vi "Recall aNETka (single).vi"() -> ()   [LabVIEW 2010]
uses:
  <vilib>/Utility/file.llb/Read From Spreadsheet File (DBL).vi
panel:
  in  "Case Constant\n(See Context Help)":bool
  out "aNETka outputs":dbl[](array[numeric])=[10.998674392700195] format="%.4f"
  out "1D config":i32[](array[numeric])=[2, 5, 1]
  out "Function":enum16{"Linear", "Sigmoid", "Tangent hyp."}(ring)=enum."Sigmoid"
  out "aNETka config":i32[](array[numeric])=[2, 5, 1] min=0 max=100 step=1
  out "aNETka configuration":cluster{dbl[], dbl[]}[](graph)=[{[2.0, 3.0], [5.5, 3.5]}, {[2.0, 3.0], [4.5, 3.5]}, {[2.0, 3.0], [3.5, 3.5]}, {[2.0, 3.0], [2.5, 3.5]}, {[2.0, 3.0], [1.5, 3.5]}, {[1.0, 2.0], [4.0, 1.5]}, {[1.0, 2.0], [4.0, 2.5]}, {[1.0, 2.0], [4.0, 3.5]}, {[1.0, 2.0], [4.0, 4.5]}, {[1.0, 2.0], [4.0, 5.5]}, {[1.0, 2.0], [3.0, 1.5]}, {[1.0, 2.0], [3.0, 2.5]}, {[1.0, 2.0], [3.0, 3.5]}, {[1.0, 2.0], [3.0, 4.5]}, {[1.0, 2.0], [3.0, 5.5]}]
  # "Inputs"
  # "Outputs"
  # "(Hidden layers)"
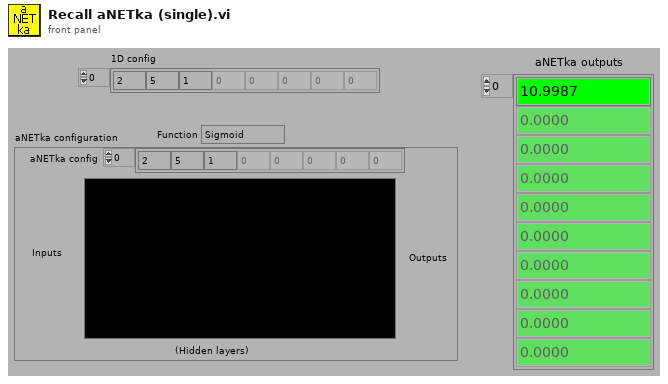
[diagram p1: front panel]
types:
  T1 = enum32{"existing file", "new file", "new or existing file", "existing dir", "new dir", "new or existing dir", "existing file (use LLBs)", "new file (use LLBs)", "new or existing file (use LLBs)", "new or existing file or directory (use LLBs)"}
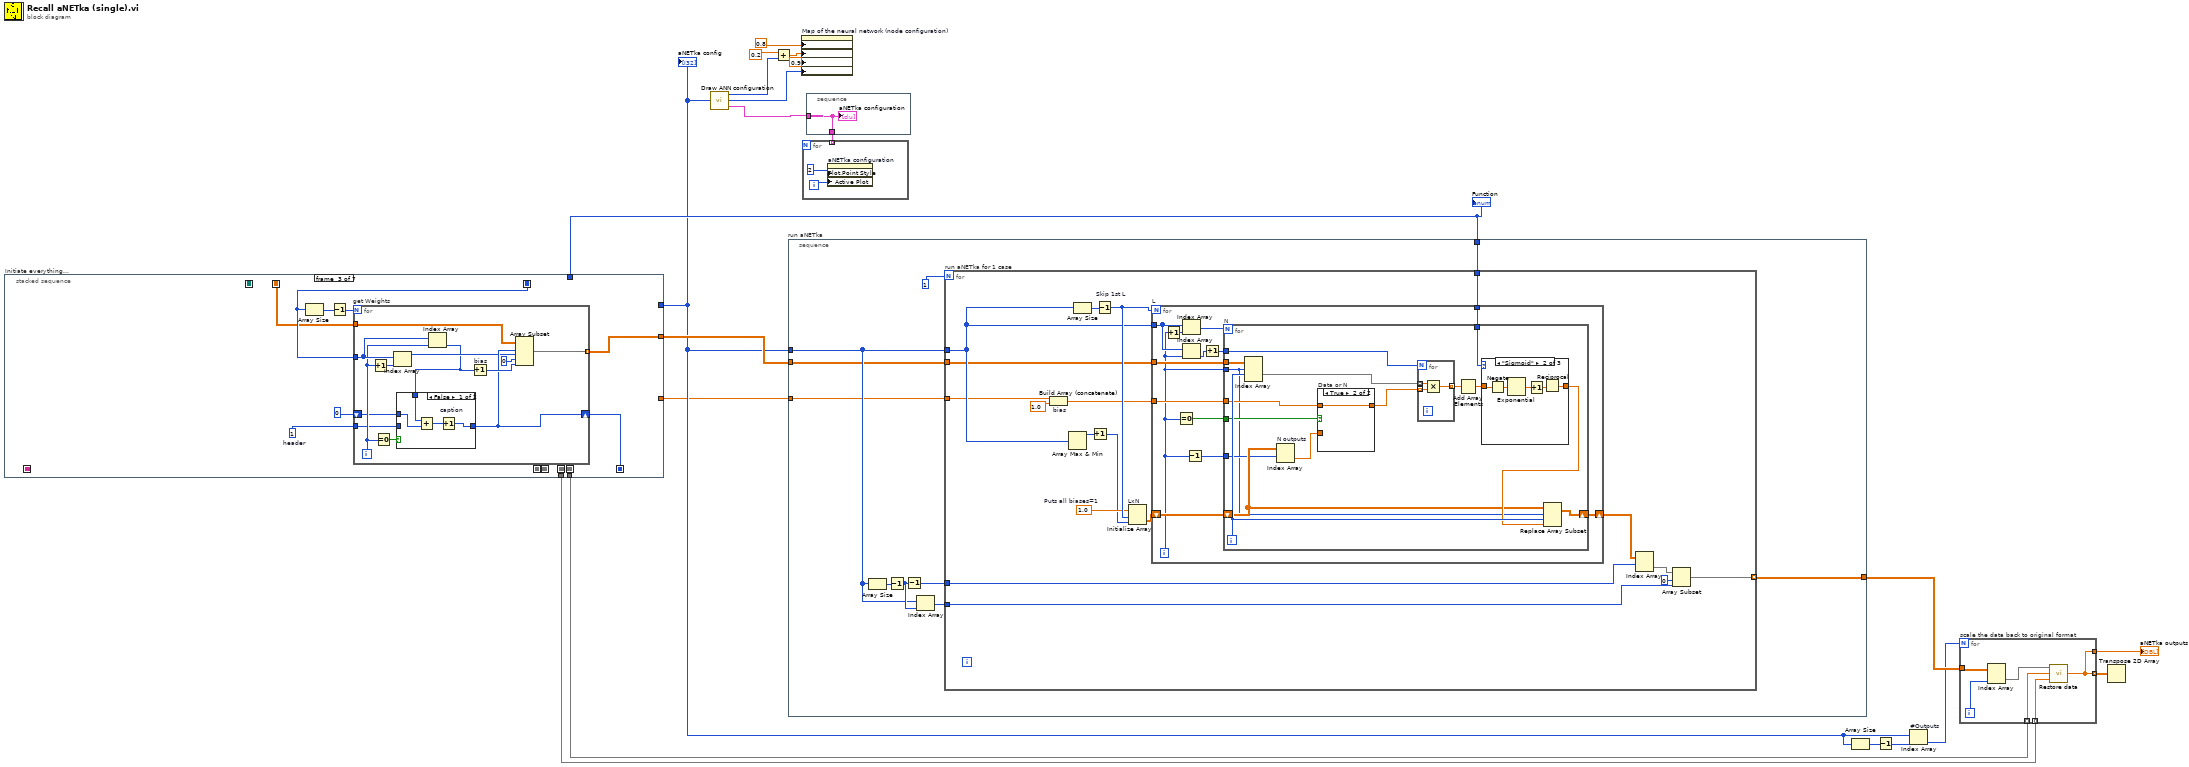
[diagram p0: block diagram]
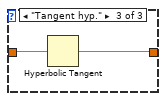
[diagram p3: hidden frame]
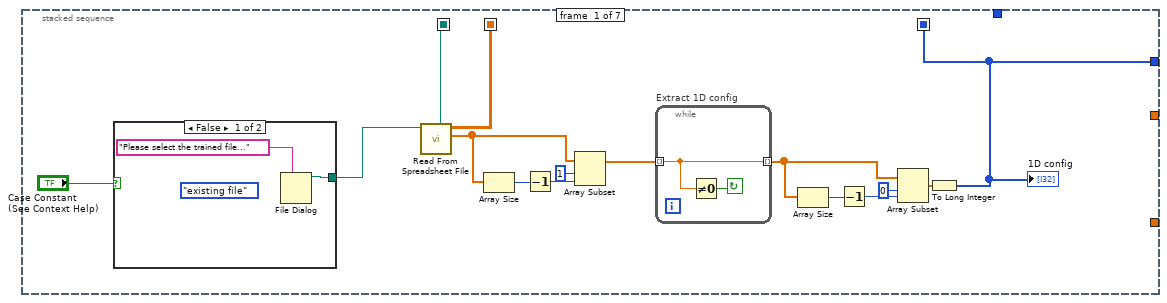
[diagram p5: hidden frame]
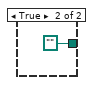
[diagram p6: hidden frame]
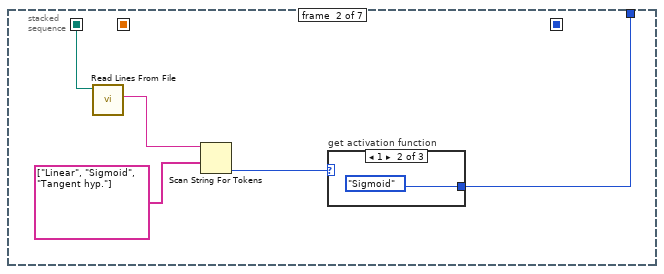
[diagram p7: hidden frame]
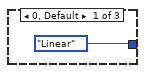
[diagram p8: hidden frame]
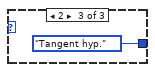
[diagram p9: hidden frame]
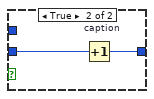
[diagram p10: hidden frame]
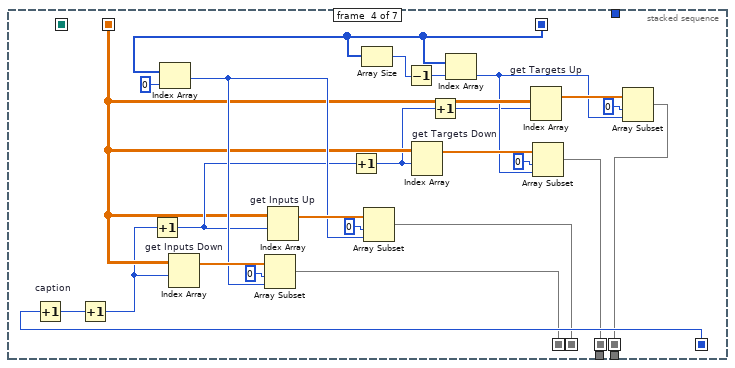
[diagram p11: hidden frame]
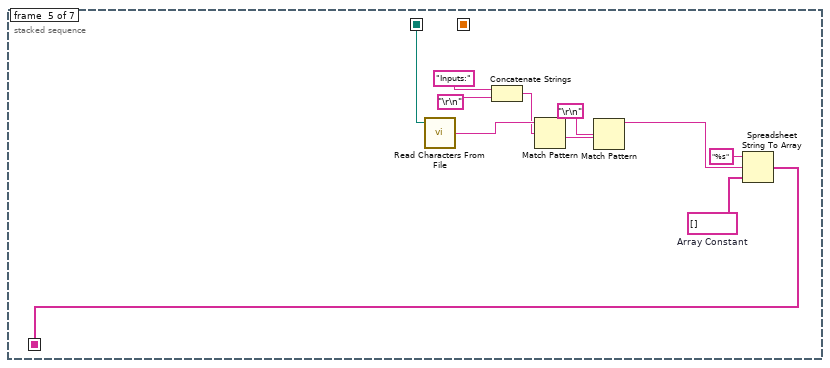
[diagram p12: hidden frame]
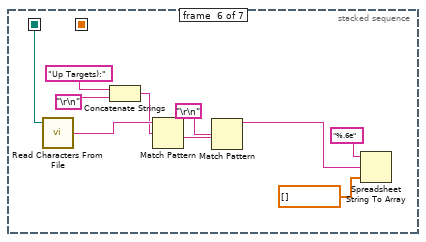
[diagram p13: hidden frame]
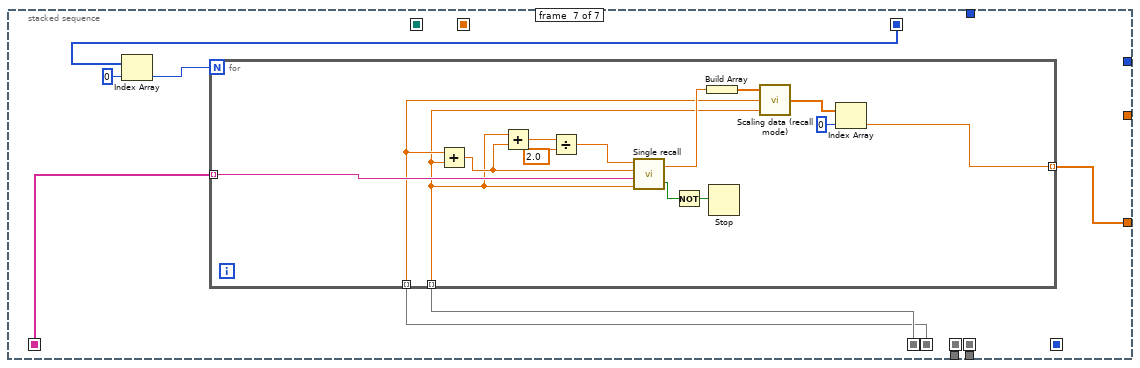
[diagram p14: hidden frame]
diagram:
  n1 = stacked-sequence "Initiate everything..." {
    seq-local: [w24 _ _ _ _ _ _] -> [_ _ w54 w89 _ _ w127]
    seq-local: [w25 _ _ _ _ _ _] -> [_ _ w53 w84 _ _ _]
    seq-local: [w23 _ _ _ _ _ _] -> [_ w45 _ _ w111 w121 _]
    seq-local: [_ _ w49 _ _ _ _] -> [_ _ _ w100 _ _ _]
    seq-local: [_ _ _ w79 _ _ _] -> [_ _ _ _ _ _ w123]
    seq-local: [_ _ _ w78 _ _ _] -> [_ _ _ _ _ _ w122]
    seq-local: [_ _ _ w76 _ _ _] -> [_ _ _ _ _ _ _]
    seq-local: [_ _ _ w77 _ _ _] -> [_ _ _ _ _ _ _]
    seq-local: [_ _ _ _ w101 _ _] -> [_ _ _ _ _ _ w125]
    tunnel: [w24 _ _ _ _ _ _] -> w5
    tunnel: [_ w41 _ _ _ _ _] -> w12
    tunnel: [_ _ w50 _ _ _ _] -> w11
    tunnel: [_ _ _ w77 _ _ _] -> w4
    tunnel: [_ _ _ w76 _ _ _] -> w3
    tunnel: [_ _ _ _ _ _ w124] -> w2
    frame #0 {
      n2 = case shown="False" "Case Constant\n(See Context Help)" {
        tunnel: [w38 path ""] -> w21
        frame False {
          (unwired) T1."existing file" ("select mode (2)")
          n3 = File Dialog(7:"Please select the trained file..." ("prompt")) -> (3:w38:path)  [unwired: 6 in, 3 out]
        }
        frame True {
        }
      }
      n4 = call-poly <vilib>:"Read From Spreadsheet File.vi"("file path (dialog if empty)"=w21) -> ("first row"=w32:dbl[], "all rows"=w25:dbl[][], "new file path (Not A Path if cancelled)"=w23:path)  [unwired: 6 in, 2 out]
      n5 = Array Size(array=w32) -> (size(s)=w34:i32)
      n6 = Decrement(x=w34) -> (x-1=w33:i32)
      n7 = Array Subset(array=w32, index=1 ("Array Index"), length=w33) -> (w31:dbl[])
      n8 = while "Extract 1D config" {
        tunnel: [w36] -> w29 mode=indexing
        tunnel: w31 -> [w36] mode=indexing
        stop <- w37 continue-if-true
        n9 = Not Equal To 0?(x=w36) -> (x != 0?=w37:bool)
      }
      n10 = Array Size(array=w29) -> (size(s)=w30:i32)
      n11 = Decrement(x=w30) -> (x-1=w28:i32)
      n12 = Array Subset(array=w29, index=0 ("Array Index"), length=w28) -> (w26:dbl[])
      n13 = To Long Integer(number=w26) -> (32bit integer=w24:i32[])
      "1D config" <- w24
    }
    frame #1 {
      n14 = call <vilib>:"Read Lines From File.vi"("file path (dialog if empty)"=w45) -> ("line string"=w44:string)  [unwired: 5 in, 3 out]
      n15 = Scan String For Tokens(7:string[] ["Linear", "Sigmoid", "Tangent hyp."] ("operators (none)"), 9:w44) -> (0:w42:i32)  [unwired: 4 in, 3 out]
      n16 = case "get activation function" shown="1" w42 {
        tunnel: [enum16{"Linear", "Sigmoid", "Tangent hyp."}."Linear" ("Function 2") enum16{"Linear", "Sigmoid", "Tangent hyp."}."Sigmoid" ("Function 2") enum16{"Linear", "Sigmoid", "Tangent hyp."}."Tangent hyp." ("Function 2")] -> w41
        frame 0, Default {
        }
        frame 1 {
        }
        frame 2 {
        }
      }
    }
    frame #2 {
      w52 = 1  # header
      n17 = Array Size(array=w54) -> (size(s)=w56:i32)
      n18 = Decrement(x=w56) -> (x-1=w55:i32)
      n19 = for "get Weights" {
        N: w55 -> [_]
        tunnel: w54 -> [w68]
        tunnel: w53 -> [w63]
        tunnel: [w62] -> w50 mode=indexing
        tunnel: w52 -> [w61]
        shift-right: [w59] -> w49
        shift-left: 0 -> [w60]
        i -> [w64]
        n20 = Increment(x=w64) -> (x+1=w69:i32)
        n21 = Equal To 0?(x=w64) -> (x = 0?=w65:bool)
        n22 = Index Array(array=w68, index=w69) -> (element=w58:i32)
        n23 = Index Array(array=w68, index=w64) -> (element=w57:i32)
        n24 = case shown="False" w65 {
          tunnel: [w71 w75] -> w59
          tunnel: w61 -> [_ w74]
          tunnel: w57 -> [w73 _]
          tunnel: w60 -> [w70 _]
          frame False {
            n25 = Add(x=w73, y=w70) -> (x+y=w72:i32)
            n26 = Increment "caption"(x=w72) -> (x+1=w71:i32)
          }
          frame True {
            n27 = Increment "caption"(x=w74) -> (x+1=w75:i32)
          }
        }
        n28 = Increment "bias"(x=w57) -> (x+1=w66:i32)
        n29 = Array Subset(array=w63, index (row)=w59, length (row)=w58, index (col)=0 ("Array Index"), length (col)=w66) -> (w62:dbl[][])
      }
    }
    frame #3 {
      n30 = Increment "caption"(x=w100) -> (x+1=w93:i32)
      n31 = Increment(x=w93) -> (x+1=w80:i32)
      n32 = Increment(x=w80) -> (x+1=w90:i32)
      n33 = Index Array(array=w89, index=0 ("Index")) -> (element=w94:i32)
      n34 = Index Array "get Inputs Down"(array=w84, index (row)=w80) -> (element=w98:dbl[])  [unwired: 1 in]
      n35 = Array Subset(array=w98, index=0 ("Array Index"), length=w94) -> (w79:dbl[])
      n36 = Index Array "get Inputs Up"(array=w84, index (row)=w90) -> (element=w95:dbl[])  [unwired: 1 in]
      n37 = Increment(x=w90) -> (x+1=w82:i32)
      n38 = Array Size(array=w89) -> (size(s)=w88:i32)
      n39 = Array Subset(array=w95, index=0 ("Array Index"), length=w94) -> (w78:dbl[])
      n40 = Decrement(x=w88) -> (x-1=w87:i32)
      n41 = Index Array "get Targets Down"(array=w84, index (row)=w82) -> (element=w91:dbl[])  [unwired: 1 in]
      n42 = Increment(x=w82) -> (x+1=w81:i32)
      n43 = Index Array(array=w89, index=w87) -> (element=w83:i32)
      n44 = Index Array "get Targets Up"(array=w84, index (row)=w81) -> (element=w86:dbl[])  [unwired: 1 in]
      n45 = Array Subset(array=w91, index=0 ("Array Index"), length=w83) -> (w76:dbl[])
      n46 = Array Subset(array=w86, index=0 ("Array Index"), length=w83) -> (w77:dbl[])
    }
    frame #4 {
      w103 = string[] []  # Array Constant
      n47 = call <vilib>:"Read Characters From File.vi"("file path (dialog if empty)"=w111) -> ("character string"=w110:string)  [unwired: 5 in, 3 out]
      n48 = Concatenate Strings("Inputs:" ("regular expression"), "\r\n") -> (w107:string)
      n49 = Match Pattern(string=w110, regular expression=w107) -> (after substring=w105:string)  [unwired: 1 in, 3 out]
      n50 = Match Pattern(string=w105, regular expression="\r\n") -> (before substring=w102:string)  [unwired: 1 in, 3 out]
      n51 = Spreadsheet String To Array(format string="%s", spreadsheet string=w102, array type (2D Dbl)=w103) -> (array=w101:string[])  [unwired: 1 in]
    }
    frame #5 {
      n52 = call <vilib>:"Read Characters From File.vi"("file path (dialog if empty)"=w121) -> ("character string"=w120:string)  [unwired: 5 in, 3 out]
      n53 = Concatenate Strings("Up Targets):" ("regular expression"), "\r\n") -> (w117:string)
      n54 = Match Pattern(string=w120, regular expression=w117) -> (after substring=w115:string)  [unwired: 1 in, 3 out]
      n55 = Match Pattern(string=w115, regular expression="\r\n") -> (before substring=w113:string)  [unwired: 1 in, 3 out]
      n56 = Spreadsheet String To Array(format string="%.6e", spreadsheet string=w113, array type (2D Dbl)=dbl[] []) -> ()  [unwired: 1 in, 1 out]
    }
    frame #6 {
      n57 = Index Array(array=w127, index=0 ("Index")) -> (element=w126:i32)
      n58 = for {
        N: w126 -> [_]
        tunnel: w125 -> [w142] mode=indexing
        tunnel: [w129] -> w124 mode=indexing
        tunnel: w123 -> [w132] mode=indexing
        tunnel: w122 -> [w133] mode=indexing
        n59 = Add(x=w133, y=w132) -> (x+y=w139:dbl)
        n60 = Add(x=w132, y=w139) -> (x+y=w138:dbl)
        n61 = Divide(x=w138, y=sgl 2.0) -> (x/y=w136:dbl)
        n62 = call "Single recall.vi"("Min limit"=w132, "Caption"=w142, "Max limit"=w139, "Input value"=w136) -> ("Continue? (T=yes)"=w140:bool, "Input value"=w134:dbl)
        n63 = Not(x=w140) -> (.not. x?=w141:bool)
        n64 = Build Array(w134) -> (w135:dbl[])
        n65 = Stop(stop? (T)=w141) -> ()
        n66 = call "Scaling data (recall mode).vi"("Offset down"=w132, "Offset up"=w133, "Input data"=w135) -> ("Scaled data"=w131:sgl[])
        n67 = Index Array(array=w131, index=0 ("Index")) -> (element=w129:sgl)
      }
    }
  }
  "aNETka config" <- w5
  "Function" <- w12
  n68 = call "Draw ANN configuration.vi"("Array"=w5) -> ("Xmax"=w20:i8, "Ymax"=w17:i16, "Map of the neural network (node configuration)"=w14:cluster{dbl[], dbl[]}[])
  n69 = Add(x=0.2, y=w20) -> (x+y=w18:dbl)
  n70 = stacked-sequence "run aNETka" {
    tunnel: w12 -> [w152]
    tunnel: w5 -> [w147]
    tunnel: w11 -> [w146]
    tunnel: [w145] -> w9
    tunnel: w2 -> [w143]
    frame #0 {
      n71 = Array Size(array=w147) -> (size(s)=w150:i32)
      n72 = Decrement(x=w150) -> (x-1=w151:i32)
      n73 = Decrement(x=w151) -> (x-1=w149:i32)
      n74 = Index Array(array=w147, index=w151) -> (element=w148:i32)
      n75 = for "run aNETka for 1 case" {
        N: 1 -> [_]
        tunnel: w147 -> [w159]
        tunnel: w152 -> [w168]
        tunnel: w149 -> [w158]
        tunnel: w148 -> [w157]
        tunnel: w146 -> [w156]
        tunnel: [w154] -> w145 mode=indexing
        tunnel: w143 -> [w155]
        w164 = sgl 1.0  # Puts all biases=1
        n76 = Build Array (concatenate) "bias"(w155, sgl 1.0 ("Input Element")) -> (w153:sgl[])
        n77 = Array Max & Min(array=w159) -> (max value=w163:i32)  [unwired: 3 out]
        n78 = Array Size(array=w159) -> (size(s)=w165:i32)
        n79 = Increment(x=w163) -> (x+1=w161:i32)
        n80 = Decrement "Skip 1st L"(x=w165) -> (x-1=w166:i32)
        n81 = Initialize Array "LxN"(w164, w166, w161) -> (w162:sgl[][])
        n82 = for "L" {
          N: w166 -> [_]
          shift-right: [w183] -> w167
          shift-left: w162 -> [w173]
          tunnel: w159 -> [w177]
          tunnel: w153 -> [w179]
          tunnel: w168 -> [w178]
          tunnel: w156 -> [w175]
          i -> [w171]
          n83 = Increment(x=w171) -> (x+1=w182:i32)
          n84 = Equal To 0?(x=w171) -> (x = 0?=w180:bool)
          n85 = Index Array(array=w177, index=w171) -> (element=w176:i32)
          n86 = Index Array(array=w177, index=w182) -> (element=w181:i32)
          n87 = Decrement(x=w171) -> (x-1=w172:i32)
          n88 = Increment(x=w176) -> (x+1=w174:i32)
          n89 = for "N" {
            N: w181 -> [_]
            shift-right: [w199] -> w183
            shift-left: w173 -> [w187]
            tunnel: w171 -> [w185]
            tunnel: w180 -> [w197]
            tunnel: w179 -> [w195]
            tunnel: w178 -> [w196]
            tunnel: w174 -> [w189]
            tunnel: w175 -> [w192]
            tunnel: w172 -> [w186]
            i -> [w198]
            n90 = Index Array(array=w192, index (dim 0)=w185, index (dim 1)=w198) -> (element=w191:dbl[])  [unwired: 1 in]
            n91 = Index Array "N outputs"(array=w187, index (row)=w186) -> (element=w190:sgl[])  [unwired: 1 in]
            n92 = case "Data or N" shown="True" w197 {
              tunnel: w190 -> [w211 _]
              tunnel: w195 -> [_ w212]
              tunnel: [w211 w212] -> w184
              frame False {
              }
              frame True {
              }
            }
            n93 = for {
              N: w189 -> [_]
              tunnel: [w202] -> w194 mode=indexing
              tunnel: w191 -> [w201] mode=indexing
              tunnel: w184 -> [w200] mode=indexing
              n94 = Multiply(x=w201, y=w200) -> (x*y=w202:dbl)
            }
            n95 = Add Array Elements(numeric array=w194) -> (sum=w193:dbl)
            n96 = case shown="\"Sigmoid\"" w196 {
              tunnel: w193 -> [w203 w205 w210]
              tunnel: [w203 w204 w209] -> w188
              frame "Linear", Default {
              }
              frame "Sigmoid" {
                n97 = Negate(x=w205) -> (-x=w208:dbl)
                n98 = Exponential(1:w208) -> (0:w207:dbl)
                n99 = Increment(x=w207) -> (x+1=w206:dbl)
                n100 = Reciprocal(x=w206) -> (1/x=w204:dbl)
              }
              frame "Tangent hyp." {
                n101 = Hyperbolic Tangent(1:w210) -> (0:w209:dbl)
              }
            }
            n102 = Replace Array Subset(array=w187, new element=w188, index (row)=w185, index (col)=w198) -> (w199:sgl[][])
          }
        }
        n103 = Index Array(array=w167, index (row)=w158) -> (element=w169:sgl[])  [unwired: 1 in]
        n104 = Array Subset(array=w169, index=0 ("Array Index"), length=w157) -> (w154:sgl[])
      }
    }
  }
  n105 = property on="Map of the neural network (node configuration)" class="XYGraph (strict)"("X Scale.Range:Minimum"=0.8, "X Scale.Range:Maximum"=w18, "Y Scale.Range:Minimum"=0.9, "Y Scale.Range:Maximum"=w17) -> ()  [unwired: 2 in, 2 out]
  n106 = stacked-sequence {
    tunnel: w14 -> [w213]
    tunnel: [w213] -> w13
    frame #0 {
      "aNETka configuration" <- w213
    }
  }
  n107 = for {
    tunnel: w13 -> [_] mode=indexing
    i -> [w214]
    n108 = property on="aNETka configuration" class="XYGraph (strict)"("Plot.Point Style"=u8 2 ("Write Attribute"), "Active Plot"=w214) -> ()  [unwired: 2 in, 2 out]
  }
  n109 = Array Size(array=w5) -> (size(s)=w8:i32)
  n110 = Decrement(x=w8) -> (x-1=w7:i32)
  n111 = Index Array "#Outputs"(array=w5, index=w7) -> (element=w6:i32)
  n112 = for "scale the data back to original format" {
    N: w6 -> [_]
    tunnel: w9 -> [w220]
    tunnel: [w216] -> w10 mode=indexing
    tunnel: w4 -> [w218] mode=indexing
    tunnel: w3 -> [w217] mode=indexing
    tunnel: [w216] -> w1
    i -> [w221]
    n113 = Index Array(array=w220, index (col)=w221) -> (element=w219:sgl[])  [unwired: 1 in]
    n114 = call "Restore data.vi"("Offset down"=w217, "Offset up"=w218, "Scaled data"=w219) -> ("Restored data"=w216:sgl[])
  }
  "aNETka outputs" <- w1
  n115 = Transpose 2D Array(2D array=w10) -> ()  [unwired: 1 out]
